vi "Settings.vi"() -> ()   [LabVIEW 2014]
panel:
  in  "Gyro Hold Integral Constant":dbl=0.03
  in  "Gyro Hold Proportionality Constant":dbl=0.03
  in  "Gyro Hold Derivative Constant":dbl=1.0
  in  "Left Back Wheel Amplification Factor":dbl=1.2
  in  "Left Front Wheel Amplification Factor":dbl=1.2
  in  "Initial Angle Uncertainty (degrees)":dbl format="%#_13g"
  in  "Initial Y Position Uncertainty (inch)":dbl format="%#_13g"
  in  "Initial X Position Uncertainty (inch)":dbl format="%#_13g"
  in  "Position Noise 4":dbl format="%#_13g"
  in  "Position Noise 3":dbl format="%#_13g"
  in  "Position Noise 2":dbl format="%#_13g"
  in  "Position Noise 1":dbl format="%#_13g"
  in  "Gyro Angle\nStd. Deviation":dbl=0.01 format="%#_13g"
  in  "Magnetometer\nStd. Deviation":dbl=0.01 format="%#_13g"
  in  "Throttle Deadband Min":dbl=-0.7
  in  "Throttle Deadband Max":dbl=0.7
  in  "Settings File Location":path=path "C:/ni-rt/startup/Settings.txt"
  in  "Swerve PID Constants":T1={"proportional gain (Kc)"=0.025, "integral time (Ti, min)"=0.0, "derivative time (Td, min)"=0.0005, "Maximum Value"=0.0005, "Minimum Value"=0.0005, "epsilon"=0.0005} {"epsilon" step=0.0001; "Minimum Value" step=0.0001; "Maximum Value" step=0.0001; "proportional gain (Kc)" step=0.01; "integral time (Ti, min)" step=0.01; "derivative time (Td, min)" step=0.0001}
  in  "Robot Twist Deadband":dbl=0.15
  in  "Robot Twist Max Value":dbl=0.75
  in  "Robot Left-RIght Deadband":dbl=0.15
  in  "Robot Left-Right Max Value":dbl=0.75
  in  "Position 1 Height (in)":dbl
  in  "Position 2 Height (in)":dbl=1.0
  in  "Position 3 Height (in)":dbl=8.0
  in  "Position 4 Height (in)":dbl=32.0625
  in  "Position 5 Height (in)":dbl=36.125
  in  "Scissors Retract Time":dbl=100.0
  in  "Scissors Extend Time":dbl=1000.0
  in  "Drawbridge Raise Tme":dbl=500.0
  in  "Drawbridge Lower Time":dbl=500.0
  in  "Arm Twister Time to Twist":dbl=1000.0
  in  "Encoder Time-Out (Lifter SS Safeties)":dbl=200.0
  in  "Default Lifter Speed":dbl=0.25
  in  "Manual Override Lifter Speed":dbl=0.25
  in  "Lifter Bump Speed Down":dbl=-0.25
  in  "Lifter Bump Speed Up":dbl=0.25
  in  "Bang-Bang Swerve Angle Deadband":dbl=9.0
  in  "Bang-Bang Swerve Twist Motor Power":dbl=0.5
  in  "Robot Forward-Reverse Deadband":dbl=0.15
  in  "Robot Forward-Reverse Max Value":dbl=0.75
  # "ms"
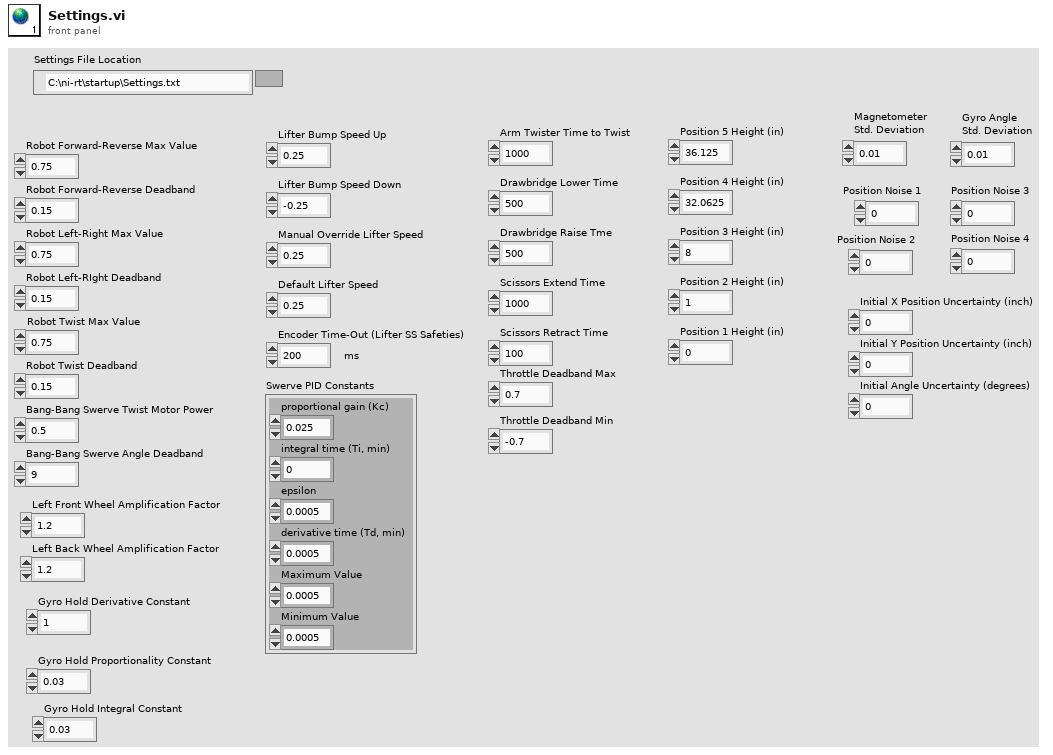
[diagram p1: front panel]
types:
  T1 = cluster{"proportional gain (Kc)":dbl, "integral time (Ti, min)":dbl, "derivative time (Td, min)":dbl, "Maximum Value":dbl, "Minimum Value":dbl, "epsilon":dbl}
diagram:
